vi "Prompt for Step--Init UI.vi"(8 "error in (no error)":errorcluster, 10 "Control Ref Map":map{string, refnum<vi>}(c390), 11 "String Assertion in":refnum<class "String Assertion.lvclass">) -> (0 "error out":errorcluster, 3 "String Assertion out":refnum<class "String Assertion.lvclass">)   [LabVIEW 2020, in "MacroAssert.lvlib" / "String Assertion.lvclass"]
doc: "Initializes the user interface within the \"Prompt for Step\" VI."
uses:
  String Assertion.lvclass
  Assertion Step/Assertion Step.lvclass
  String Assertion.lvclass/String Assertion.ctl
  MacroAssert.lvlib
  Support/Get Control Reference by Label (1D STR).vi
  52795b1d-0798-46ad-a109-a5c41e831e76.vi
  55d5fdb2-f8b0-48c8-993e-5734b642cc86.vi
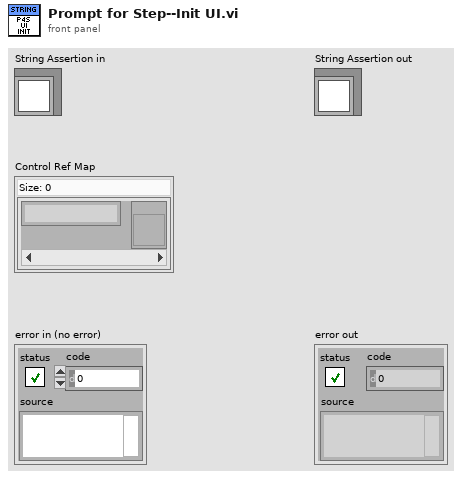
[diagram p1: front panel]
types:
  T1 = typedef "MacroAssert.lvlib/String Assertion.lvclass/String Assertion Type.ctl" = enum16{"String Ctl Value", "Ctl Caption Property", "Ctl Tip Strip Property", "Frontmost VI Name", "Frontmost Window Name"}
  T2 = typedef "MacroAssert.lvlib/String Assertion.lvclass/String Comparator.ctl" = enum16{"Contains", "Equals", "Starts with", "Ends with", "Does not contain", "Does not equal"}
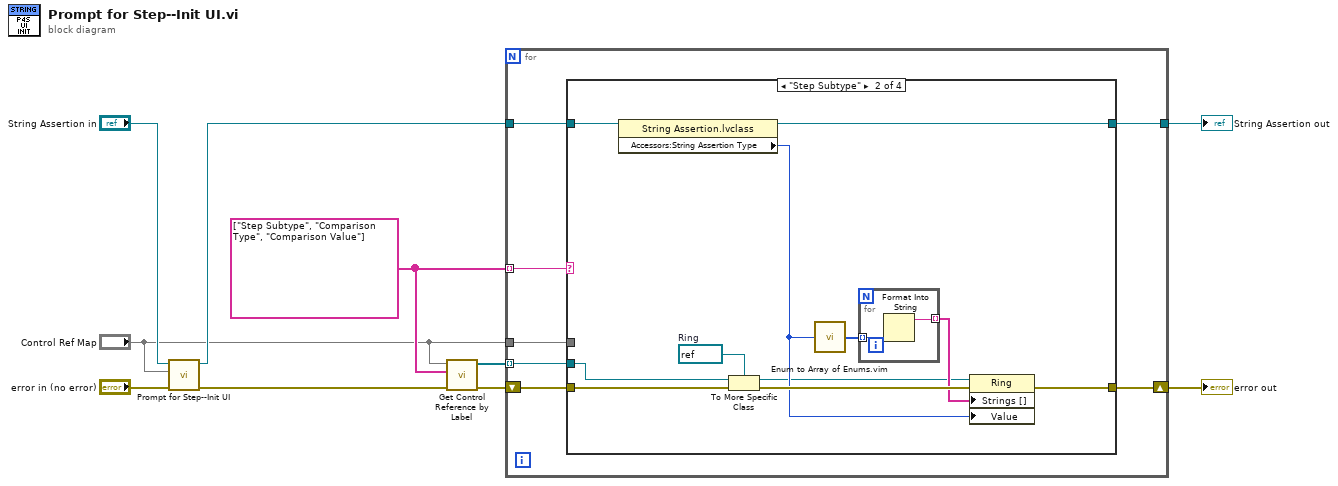
[diagram p0: block diagram]
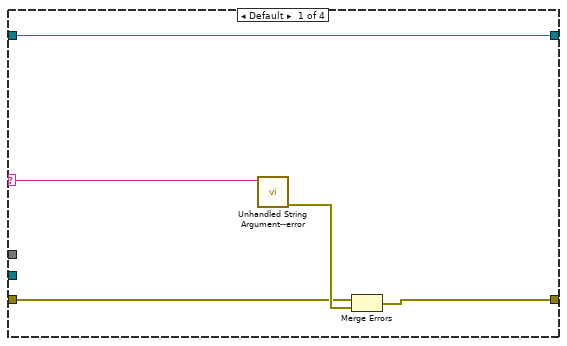
[diagram p2: hidden frame]
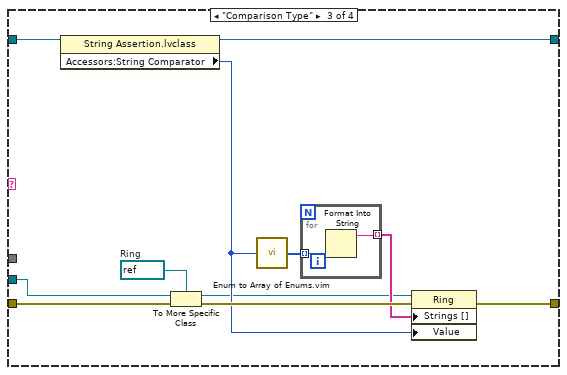
[diagram p3: hidden frame]
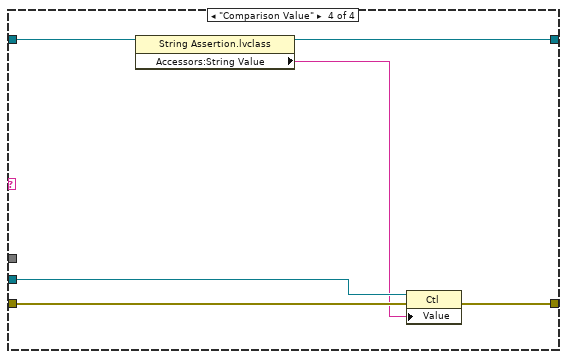
[diagram p4: hidden frame]
diagram:
  w9 = string[] ["Step Subtype", "Comparison Type", "Comparison Value"]
  n1 = call-parent "Prompt for Step--Init UI.vi"("error in (no error)"="error in (no error)", "Control Ref Map"="Control Ref Map", "Assertion Step in"="String Assertion in") -> ("error out"=w4:errorcluster, "Assertion Step out"=w2:refnum<class "String Assertion.lvclass">)  [unwired: 7 in]
  n2 = call-poly "Get Control Reference by Label.vi"("error in (no error)"=w4, "Control Names"=w9, "Control Ref Map"="Control Ref Map") -> ("error out"=w10:errorcluster, "Control Refs"=w8:refnum<vi>[])  [unwired: 6 in, 1 out]
  n3 = for {
    tunnel: w2 -> [w15]
    tunnel: [w13] -> w6
    tunnel: w9 -> [w16] mode=indexing
    tunnel: w8 -> [w14] mode=indexing
    shift-right: [w12] -> w7
    shift-left: w10 -> [w17]
    tunnel: "Control Ref Map" -> [w11]
    n4 = case shown="\"Step Subtype\"" w16 {
      selector: w16 -> [w19 _ _ _]
      tunnel: w17 -> [w21 w26 w39 w51]
      tunnel: w15 -> [w18 w27 w40 w54]
      tunnel: w14 -> [_ w25 w38 w52]
      tunnel: [w18 w24 w37 w53] -> w13
      tunnel: [w20 w23 w36 w49] -> w12
      tunnel: w11 -> [_ _ _ _]
      frame Default {
        n5 = call "Unhandled String Argument--error.vi"("Argument"=w19) -> ("error out"=w22:errorcluster)  [unwired: 10 in]
        n6 = Merge Errors(w21, w22) -> (w20:errorcluster)
      }
      frame "Step Subtype" {
        w31 = refnum<vi> refnum  # Ring
        n7 = property class="String Assertion.lvclass"(reference=w27) -> (reference out=w24:refnum<class "String Assertion.lvclass">, "Accessors:String Assertion Type"=w30:T1)  [unwired: 1 in, 1 out]
        n8 = To More Specific Class(target class=w31, reference=w25, error in=w26) -> (specific class reference=w28:refnum<vi>, error out=w32:errorcluster)
        n9 = call "Enum to Array of Enums.vim"("enum"=w30) -> ("array of enums"=w33:T1[])
        n10 = for {
          tunnel: w33 -> [w35] mode=indexing
          tunnel: [w34] -> w29 mode=indexing
          n11 = Format Into String(w35) -> (resulting string=w34:string)  [unwired: 3 in, 1 out]
        }
        n12 = property class="Ring"(reference=w28, error in=w32, "Strings []"=w29, "Value"=w30) -> (error out=w23:errorcluster)  [unwired: 1 out]
      }
      frame "Comparison Type" {
        w44 = refnum<vi> refnum  # Ring
        n13 = property class="String Assertion.lvclass"(reference=w40) -> (reference out=w37:refnum<class "String Assertion.lvclass">, "Accessors:String Comparator"=w43:T2)  [unwired: 1 in, 1 out]
        n14 = To More Specific Class(target class=w44, reference=w38, error in=w39) -> (specific class reference=w41:refnum<vi>, error out=w45:errorcluster)
        n15 = call "Enum to Array of Enums.vim"("enum"=w43) -> ("array of enums"=w46:T2[])
        n16 = for {
          tunnel: w46 -> [w48] mode=indexing
          tunnel: [w47] -> w42 mode=indexing
          n17 = Format Into String(w48) -> (resulting string=w47:string)  [unwired: 3 in, 1 out]
        }
        n18 = property class="Ring"(reference=w41, error in=w45, "Strings []"=w42, "Value"=w43) -> (error out=w36:errorcluster)  [unwired: 1 out]
      }
      frame "Comparison Value" {
        n19 = property class="String Assertion.lvclass"(reference=w54) -> (reference out=w53:refnum<class "String Assertion.lvclass">, "Accessors:String Value"=w50:string)  [unwired: 1 in, 1 out]
        n20 = property class="Ctl"(reference=w52, error in=w51, "Value"=w50) -> (error out=w49:errorcluster)  [unwired: 1 out]
      }
    }
  }
  "error out" <- w7
  "String Assertion out" <- w6
